vi "矩形居中（TB）.vi"(10 "边界矩形":T1, 11 "矩形":T1) -> (3 "居中后的矩形":T1)   [LabVIEW 2011]
uses:
  RectTB.ctl
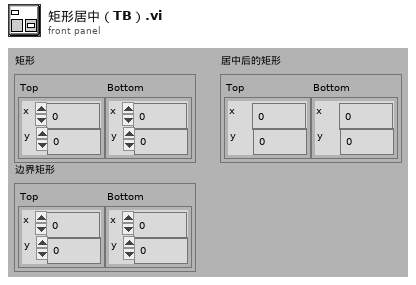
[diagram p1: front panel]
types:
  T1 = typedef "RectTB.ctl" = cluster{"Top":cluster{"x":i16, "y":i16}, "Bottom":cluster{"x":i16, "y":i16}}
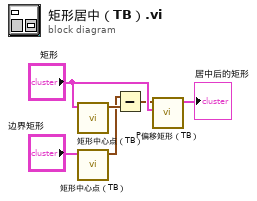
[diagram p0: block diagram]
diagram:
  n1 = call "矩形中心点（TB）.vi"("矩形"="矩形") -> ("中心点"=w5:cluster{"x":i16, "y":i16})  [unwired: 10 in]
  n2 = call "矩形中心点（TB）.vi"("矩形"="边界矩形") -> ("中心点"=w4:cluster{"x":i16, "y":i16})  [unwired: 10 in]
  n3 = Subtract(x=w4, y=w5) -> (x-y=w2:cluster{"x":i16, "y":i16})
  n4 = call "P偏移矩形（TB）.vi"("RectTB"="矩形", "point"=w2) -> ("RectTB(Offset)"=→"居中后的矩形":T1)  [unwired: 9 in]
